vi "CheckFloatSwitch.vi"(8 "error in":errorcluster) -> (0 "error out":errorcluster, 1 "Tweet text":string, 2 "Low?":bool, 3 "High?":bool)   [LabVIEW 2014]
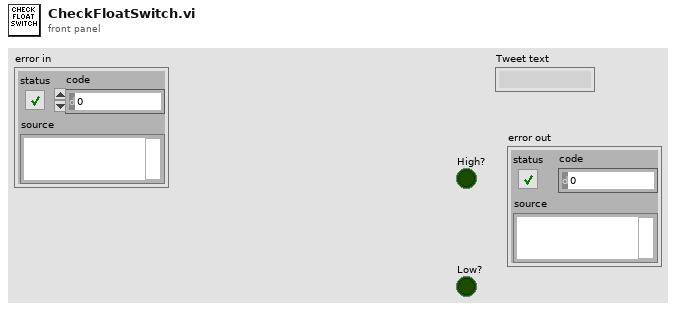
[diagram p1: front panel]
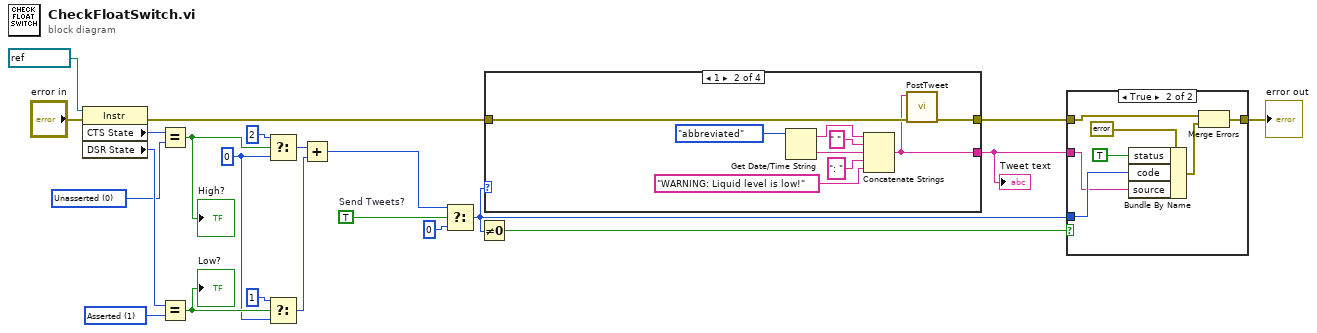
[diagram p0: block diagram]
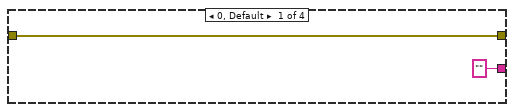
[diagram p3: hidden frame]
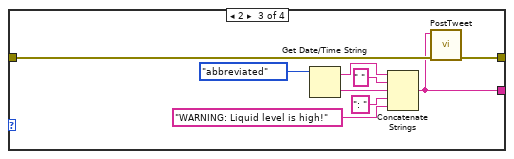
[diagram p4: hidden frame]
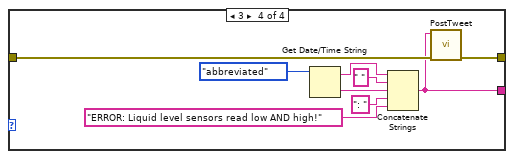
[diagram p5: hidden frame]
diagram:
  w1 = i16 0 items=["Unknown"=-1, "Unasserted"=0, "Asserted"=1] ("Serial Settings:Modem Line Settings:Line DSR State 2")
  w9 = TRUE  # Send Tweets?
  w14 = u8 0 ("f")
  w20 = i16 1 items=["Unknown"=-1, "Unasserted"=0, "Asserted"=1] ("Serial Settings:Modem Line Settings:Line DSR State 2")
  n1 = property class="Instr"(reference=refnum<visa-resource-name> "COM1" ("VISA resource name"), error in="error in") -> (error out=w18:errorcluster, "CTS State"=w21:i16, "DSR State"=w22:i16)  [unwired: 1 out]
  n2 = Equal?(x=w21, y=w1) -> (x = y?=w17:bool)
  "High?" <- w17
  n3 = Equal?(x=w22, y=w20) -> (x = y?=w15:bool)
  "Low?" <- w15
  n4 = Select(t=u8 2 ("f"), s=w17, f=w14) -> (s? t:f=w11:u8)
  n5 = Select(t=u8 1 ("f"), s=w15, f=w14) -> (s? t:f=w12:u8)
  n6 = Add(x=w11, y=w12) -> (x+y=w10:u8)
  n7 = Select(t=w10, s=w9, f=u8 0) -> (s? t:f=w6:u8)
  n8 = Not Equal To 0?(x=w6) -> (x != 0?=w7:bool)
  n9 = case shown="1" w6 {
    tunnel: w18 -> [w24 w33 w41 w51]
    tunnel: [w24 w32 w42 w50] -> w3
    tunnel: ["" w30 w39 w44] -> w5
    frame 0, Default {
    }
    frame 1 {
      n10 = Get Date/Time String(date format (0)=enum16{"short", "long", "abbreviated"}."abbreviated") -> (date string=w31:string, time string=w28:string)  [unwired: 2 in]
      n11 = Concatenate Strings(w31, " " ("string"), w28, ": " ("string"), "WARNING: Liquid level is low!" ("Tweet")) -> (w30:string)
      n12 = call "PostTweet.vi"("error in"=w33, "Tweet"=w30) -> ("error out"=w32:errorcluster)  [unwired: 9 in]
    }
    frame 2 {
      n13 = Get Date/Time String(date format (0)=enum16{"short", "long", "abbreviated"}."abbreviated") -> (date string=w40:string, time string=w36:string)  [unwired: 2 in]
      n14 = Concatenate Strings(w40, " " ("string"), w36, ": " ("string"), "WARNING: Liquid level is high!" ("Tweet")) -> (w39:string)
      n15 = call "PostTweet.vi"("error in"=w41, "Tweet"=w39) -> ("error out"=w42:errorcluster)  [unwired: 9 in]
    }
    frame 3 {
      n16 = Get Date/Time String(date format (0)=enum16{"short", "long", "abbreviated"}."abbreviated") -> (date string=w46:string, time string=w49:string)  [unwired: 2 in]
      n17 = Concatenate Strings(w46, " " ("string"), w49, ": " ("string"), "ERROR: Liquid level sensors read low AND high!" ("Tweet")) -> (w44:string)
      n18 = call "PostTweet.vi"("error in"=w51, "Tweet"=w44) -> ("error out"=w50:errorcluster)  [unwired: 9 in]
    }
  }
  "Tweet text" <- w5
  n19 = case shown="True" w7 {
    tunnel: w6 -> [_ w57]
    tunnel: w5 -> [_ w56]
    tunnel: [w52 w54] -> w4
    tunnel: w3 -> [w52 w55]
    frame False {
    }
    frame True {
      n20 = Bundle By Name(cluster=errorcluster {"status"=FALSE, "code"=0, "source"=""} ("error constant"), "status"=TRUE, "code"=w57, "source"=w56) -> (w53:errorcluster)
      n21 = Merge Errors(w55, w53) -> (w54:errorcluster)
    }
  }
  "error out" <- w4
